vi "Delete configuration item.vi"(7 "table name":string, 8 "error in (no error)":errorcluster, 10 "configuration item":string, 11 "IConfigDBQueries in":refnum<class "IConfigurationDatabaseQueries.lvclass">) -> (0 "error out":errorcluster)   [LabVIEW 2020, in "configuration-database.lvlib" / "IConfigurationDatabaseQueries.lvclass"]
uses:
  IConfigurationDatabaseQueries.lvclass
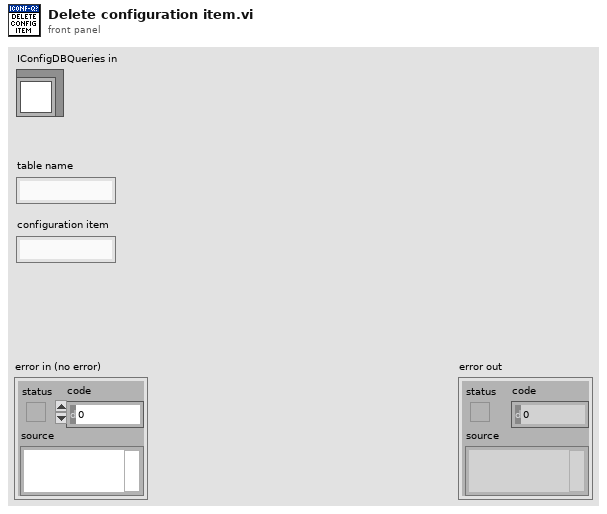
[diagram p1: front panel]
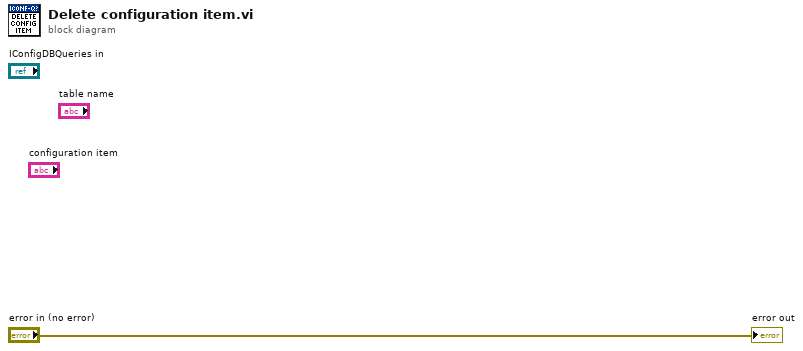
[diagram p0: block diagram]
diagram:
  "error out" <- "error in (no error)"
